vi "Probability Density Function Estimation.vi"() -> ()   [LabVIEW 2023]
doc: "This example shows how to estimate a smooth probability density function (PDF) of a signal with the WA Probability Density Function Estimation VI. This example generates a Gaussian white noise and runs tests on this white noise. You also can obtain a smooth PDF by averaging the histogram but you need more data samples.\n\n<b>Instructions:</b>\n1) Run this VI.\n2) Compare the estimated PDF of the signal with the wavelet transform-based method and the averaged-histogram method.\n3) Increase the value of the <b>Number of Histogram to Average</b>. Notice that the result of the averaged-histogram method becomes close to that of the wavelet transform-based method."
uses:
  <vilib>/addons/Wavelet Analysis/application.llb/WA Probability Density Function Estimation (1D Array).vi
  <vilib>/addons/_Advanced Signal Processing/NI_AdvSigProcWA.lvlib
  <vilib>/Analysis/NI_AALPro.lvlib
  <vilib>/Analysis/NI_AALBase.lvlib
panel:
  in  "stop":bool
  in  "Number of histogram \nto average":i32=1
  in  "Wavelet":u16(ring)=7 items=["db02"=0, "db03"=1, "db04"=2, "db05"=3, "db06"=4, "db07"=5, "db08"=6, "db09"=7, "db10"=8, "db11"=9, "db12"=10, "db13"=11, "db14"=12, "Haar"=13, "bior1_3"=14, "bior1_5"=15, "bior2_2"=16, "bior2_4"=17, "bior2_6"=18, "bior2_8"=19, "bior3_1"=20, "bior3_3"=21, "bior3_5"=22, "bior3_7"=23, "bior3_9"=24, "bior4_4 (FBI)"=25, "bior5_5"=38, "bior6_8"=39, "coif1"=26, "coif2"=27, "coif3"=28, "coif4"=29, "coif5"=30, "sym2"=31, "sym3"=32, "sym4"=33, "sym5"=34, "sym6"=35, "sym7"=36, "sym8"=37]
  out "Signal":dbl[](graph)
  out "Probability Density Function":cluster{"Axis":dbl[], dbl[]}[](graph)
  # "Overview: Shows how to estimate a smooth probability density function (PDF) of a signal with the WA Probability Density Function Estimation VI. \nRequirements: LabVIEW Full Development System, Advanced Signal Processing Toolkit\nInstructions: \n1. Run this VI.\n2. Compare the estimated PDF of the signal with the wavelet transform-based method and the averaged-histogram method.\n3. Increase the value of the Number of Histogram to Average. Notice that the result of the averaged-histogram method becomes close to that of the wavelet transform-based method.\n4. Click Stop to stop the VI."
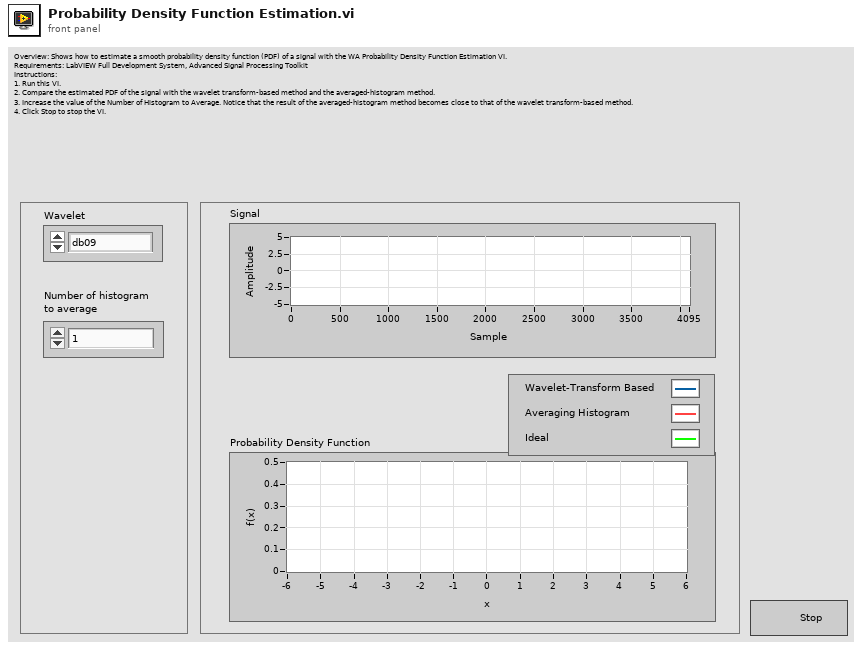
[diagram p1: front panel]
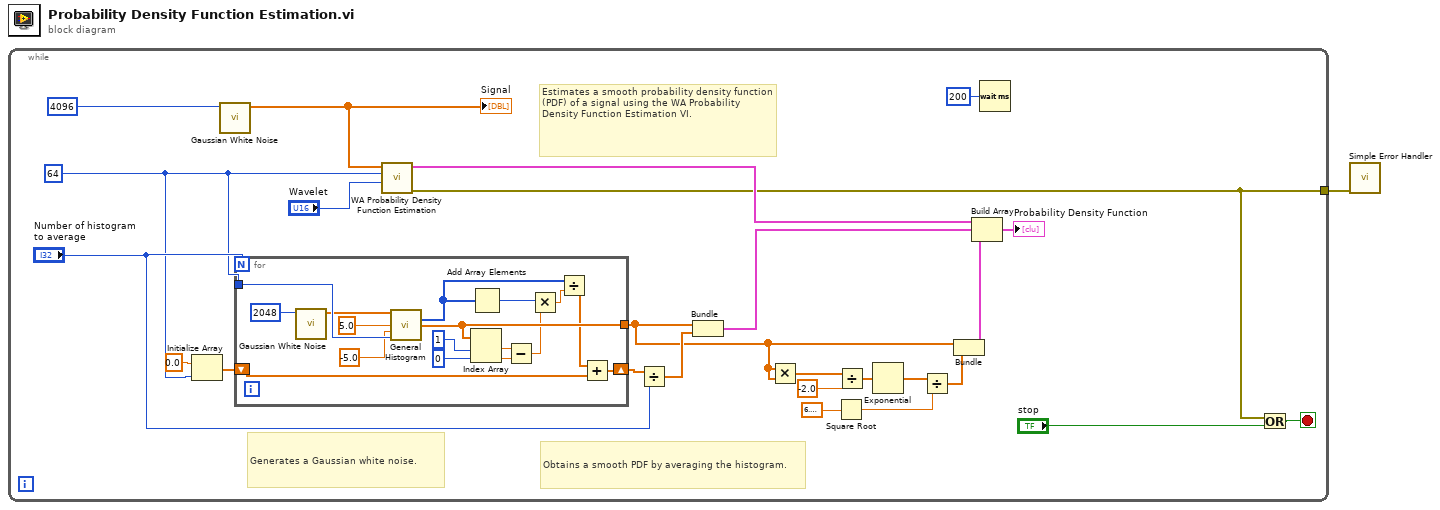
[diagram p0: block diagram]
diagram:
  n1 = while {
    tunnel: [w2] -> w1
    stop <- w6 stop-if-true
    w15 = 64 ("bin #")
    # "Obtains a smooth PDF by averaging the histogram."
    # "Generates a Gaussian white noise."
    # "Estimates a smooth probability density function (PDF) of a signal using the WA Probability Density Function Estimation VI."
    n2 = Initialize Array(0.0 ("element"), w15) -> (w17:dbl[])
    n3 = call <vilib>:"Gaussian White Noise.vi"("samples"=4096) -> ("Gaussian noise pattern"=w24:dbl[])  [unwired: 9 in, 1 out]
    "Signal" <- w24
    n4 = for {
      N: "Number of histogram \nto average" -> [_]
      tunnel: w15 -> [w43]
      tunnel: [w35] -> w8
      shift-right: [w39] -> w20
      shift-left: w17 -> [w40]
      n5 = call <vilib>:"Gaussian White Noise.vi"("samples"=2048) -> ("Gaussian noise pattern"=w41:dbl[])  [unwired: 9 in, 1 out]
      n6 = call <vilib>:"General Histogram.vi"("X"=w41, "max"=5.0, "min"=-5.0, "# bins"=w43) -> ("Histogram"=w36:i32[], "Axis"=w35:dbl[])  [unwired: 2 in, 8 out]
      n7 = Index Array(array=w35, index #1=1 ("index"), index #2=0 ("index")) -> (element #1=w32:dbl, element #2=w31:dbl)
      n8 = Add Array Elements(numeric array=w36) -> (sum=w30:i32)
      n9 = Subtract(x=w32, y=w31) -> (x-y=w29:dbl)
      n10 = Multiply(x=w30, y=w29) -> (x*y=w28:dbl)
      n11 = Divide(x=w36, y=w28) -> (x/y=w27:dbl[])
      n12 = Add(x=w27, y=w40) -> (x+y=w39:dbl[])
    }
    n13 = call-poly <vilib>:"WA Probability Density Function Estimation.vi"("wavelet"="Wavelet", "number of bins"=w15, "signal"=w24) -> ("error out"=w2:errorcluster, "PDF"=w23:cluster{"Axis":dbl[], dbl[]})  [unwired: 1 in, 6 out]
    n14 = Divide(x=w20, y="Number of histogram \nto average") -> (x/y=w19:dbl[])
    n15 = Bundle("Axis"=w8, w19) -> (w21:cluster{"Axis":dbl[], dbl[]})  [unwired: 1 out]
    n16 = Multiply(x=w8, y=w8) -> (x*y=w14:dbl[])
    n17 = Square Root(x=6.283185307179586 ("Pi Multiplied By 2")) -> (sqrt(x)=w4:dbl)
    n18 = Divide(x=w14, y=-2.0) -> (x/y=w13:dbl[])
    n19 = Exponential(1:w13) -> (0:w11:dbl[])
    n20 = Divide(x=w11, y=w4) -> (x/y=w10:dbl[])
    n21 = Bundle("Axis"=w8, w10) -> (w9:cluster{"Axis":dbl[], dbl[]})  [unwired: 1 out]
    n22 = Build Array(w23, w21, w9) -> (→"Probability Density Function":cluster{"Axis":dbl[], dbl[]}[])
    n23 = Wait (ms)(milliseconds to wait=u32 200 ("millisecond multiple")) -> ()  [unwired: 1 out]
    n24 = Or(x=w2, y="stop") -> (x .or. y?=w6:bool)
  }
  n25 = call <vilib>:"Simple Error Handler.vi"("error in (no error)"=w1) -> ()  [unwired: 1 in, 8 out]
